vi "Msg.vi"(7 "Actor in":refnum<class "Actor.lvclass">, 11 "Last Ack Msg in":refnum<class "Last Ack Msg.lvclass">) -> (5 "Actor out":refnum<class "Actor.lvclass">)   [LabVIEW 2021, in "Last Ack.lvlib" / "Last Ack Msg.lvclass"]
uses:
  Last Ack Msg.lvclass
  jettl/Actor/Actor.lvclass
  Last Ack/Last Ack.lvclass
  26d28521-7f61-4032-a412-881153c4d1f0.vi
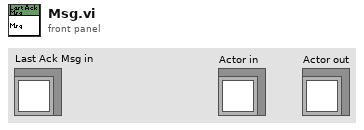
[diagram p1: front panel]
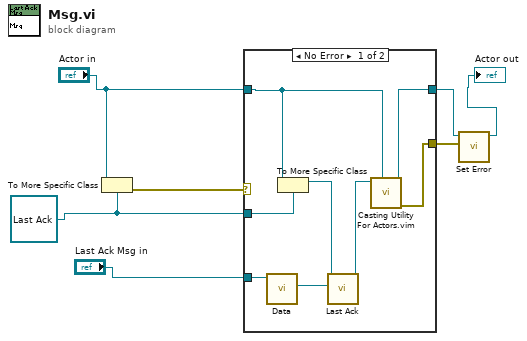
[diagram p0: block diagram]
diagram:
  w4 = refnum<class "Last Ack.lvclass"> refnum ("Last Ack.lvlib:Last Ack.lvclass")
  n1 = To More Specific Class(target class=w4, reference="Actor in") -> (error out=w7:errorcluster)  [unwired: 1 in, 1 out]
  n2 = case shown="No Error" w7 {
    selector: w7 -> [_ w16]
    tunnel: [w14 w17] -> w3
    tunnel: "Actor in" -> [w13 w17]
    tunnel: w4 -> [w15 _]
    tunnel: "Last Ack Msg in" -> [w12 _]
    tunnel: [w8 w16] -> w1
    frame No Error {
      n3 = call "Data.vi"("Last Ack Msg in"=w12) -> ("Actor"=w9:refnum<class "Actor.lvclass">)  [unwired: 10 in]
      n4 = To More Specific Class(target class=w15, reference=w13) -> (specific class reference=w10:refnum<class "Last Ack.lvclass">)  [unwired: 1 in, 1 out]
      n5 = call-dynamic "Last Ack.vi"("Actor"=w9, "Last Ack in"=w10) -> ("Last Ack out"=w11:refnum<class "Last Ack.lvclass">)  [unwired: 9 in]
      n6 = call "Casting Utility For Actors.vim"("type"=w13, "Actor in"=w11) -> ("error out"=w8:errorcluster, "Actor out"=w14:refnum<class "Actor.lvclass">)  [unwired: 8 in]
    }
    frame Error {
    }
  }
  n7 = call-dynamic "Set Error.vi"("Error"=w1, "Actor in"=w3) -> ("Actor out"=→"Actor out":refnum<class "Actor.lvclass">)  [unwired: 9 in]
